vi "DAQ Analog Out.Async.vi"(10 "Parameters":variant, 11 "Process":refnum<class "Process.lvclass">) -> ()   [LabVIEW 2021, in "DAQ Analog InOut Engine.lvlib"]
uses:
  DAQ Analog InOut Engine.lvlib
  <vilib>/NI/NIVS Inline Async API/_VS Inline Async API/Process/Process.lvclass
  AO Properties.ctl
  System Explorer/Types/Output Channel Parameters.ctl
  <vilib>/NI/NIVS Inline Async API/_VS Inline Async API/Process/Process.lvclass/Process.ctl
  <vilib>/NI/NIVS Inline Async API/_Data Access Engine/Access Type Classes/Read/Read.lvclass/Read.ctl
  <vilib>/NI/NIVS Inline Async API/_Data Access Engine/Data Access Engine/Methods/Read.Data.vi
  <vilib>/DAQmx/write.llb/DAQmx Write (Analog 1D DBL NChan 1Samp).vi
  <vilib>/NI/NIVS Inline Async API/_VS Inline Async API/Process/Data Member Access/Read Data Access.vi
  <vilib>/NI/NIVS Inline Async API/_VS Inline Async API/Error Handling Process/SubVIs/Error.ConvertArray.vi
  <vilib>/NI/NIVS Inline Async API/_Data Access Engine/Access Type Classes/Read/Read.ProcessData.vi
  <vilib>/NI/NIVS Inline Async API/_Data Access Engine/Data Access Engine/Methods/Read.Lookup.vi
  <vilib>/DAQmx/miscellaneous.llb/DAQmx Fill In Error Info.vi
  <vilib>/NI/NIVS Inline Async API/_Data Access Engine/Data Access Engine/Data Access Engine.lvclass
  System Explorer/DAQ Analog InOut System Explorer.lvlib
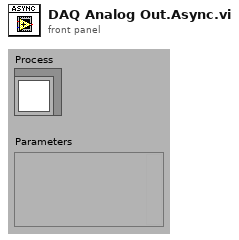
[diagram p1: front panel]
types:
  T1 = typedef "DAQ Analog InOut Engine.lvlib/AO Properties.ctl" = cluster{"AO Channels List":string, "Output Channel Parameters":T2}
  T2 = typedef "DAQ Analog InOut System Explorer.lvlib/Output Channel Parameters.ctl" = cluster{"AO MaxV":dbl, "AO MinV":dbl}
  T3 = typedef "Data Access Engine.lvlib/Data Access Engine.lvclass/Read.DVR.ctl" = refnum<data-value>
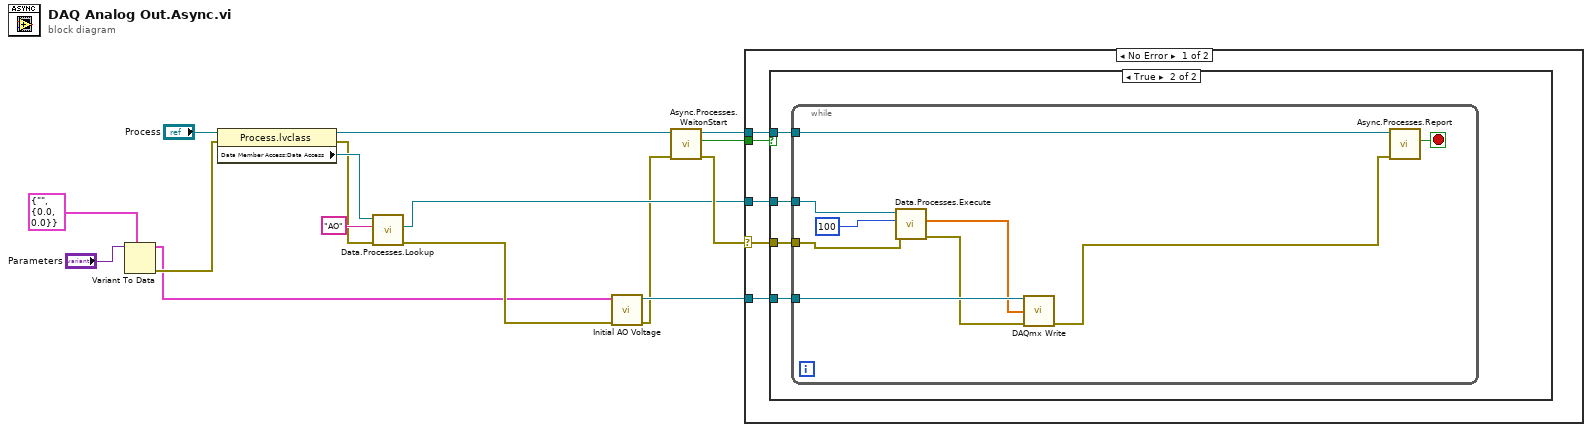
[diagram p0: block diagram]
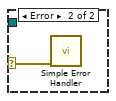
[diagram p3: hidden frame]
diagram:
  n1 = Variant To Data(type=T1 {"AO Channels List"="", "Output Channel Parameters"={"AO MaxV"=0.0, "AO MinV"=0.0}} ("AO Properties"), Variant="Parameters") -> (data=w3:T1, error out=w5:errorcluster)  [unwired: 1 in]
  n2 = property class="Process.lvclass"(reference="Process", error in=w5) -> (reference out=w10:refnum<class "Process.lvclass">, error out=w8:errorcluster, "Data Member Access:Data Access"=w9:refnum<class "Data Access Engine.lvclass">)
  n3 = call-poly <vilib>:"Data.Processes.Lookup.vi"("error in (no error)"=w8, "Name"="AO", "Data Access API in"=w9) -> ("error out"=w4:errorcluster, "Ref"=w12:T3)  [unwired: 5 in, 2 out]
  n4 = call "Initial AO Voltage.vi"("error in"=w4, "AO Properties"=w3) -> ("error out"=w1:errorcluster, "DAQ Ref out"=w2:refnum<k21>)  [unwired: 8 in]
  n5 = call <vilib>:"Async.Processes.WaitonStart.vi"("error in (no error)"=w1, "Process"=w10) -> ("error out"=w14:errorcluster, "Execute"=w16:bool, "Process out"=w15:refnum<class "Process.lvclass">)  [unwired: 7 in]
  n6 = case shown="No Error" w14 {
    selector: w14 -> [w18 w35]
    tunnel: w16 -> [w21 _]
    tunnel: w15 -> [w20 _]
    tunnel: w12 -> [w19 _]
    tunnel: w2 -> [w17 _]
    frame No Error {
      n7 = case shown="True" w21 {
        tunnel: w18 -> [_ w23]
        tunnel: w20 -> [_ w24]
        tunnel: w19 -> [_ w25]
        tunnel: w17 -> [_ w22]
        frame False {
        }
        frame True {
          n8 = while {
            tunnel: w23 -> [w30]
            tunnel: w24 -> [w34]
            tunnel: w25 -> [w32]
            tunnel: w22 -> [w29]
            stop <- w33 stop-if-true
            n9 = call-poly <vilib>:"Data.Processes.Execute.vi"("error in (no error)"=w30, "timeout ms"=100, "Ref"=w32) -> ("error out"=w28:errorcluster, "Values"=w27:dbl[])  [unwired: 6 in, 1 out]
            n10 = call-poly <vilib>:"DAQmx Write.vi"("task/channels in"=w29, "data"=w27, "error in"=w28) -> ("error out"=w26:errorcluster)  [unwired: 10 in, 2 out]
            n11 = call <vilib>:"Async.Processes.Report.vi"("Error"=w26, "Process in"=w34) -> ("Stop"=w33:bool)  [unwired: 8 in, 1 out]
          }
        }
      }
    }
    frame Error {
      n12 = call <vilib>:"Simple Error Handler.vi"("error in (no error)"=w35) -> ()  [unwired: 4 in, 5 out]
    }
  }
